vi "Unflatten LIDAR Data.vi"(11 "Flat LIDAR Data":dbl[](array[numeric])) -> (0 "Robot Pose x,y (m)":dbl[](array[numeric]), 1 "Robot Pose Theta (rad)":dbl, 2 "Bearing (rad)":dbl[](array[numeric]), 3 "Range (m)":dbl[](array[numeric]))   [LabVIEW 2017]
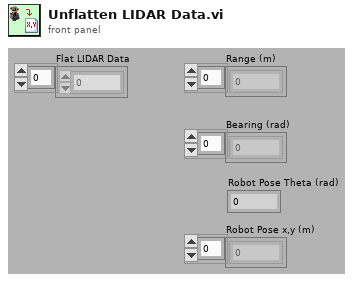
[diagram p1: front panel]
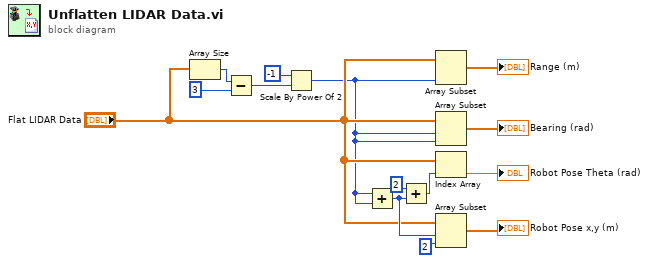
[diagram p0: block diagram]
diagram:
  n1 = Array Size(array="Flat LIDAR Data") -> (size(s)=w1:i32)
  n2 = Subtract(x=w1, y=3) -> (x-y=w3:i32)
  n3 = Scale By Power Of 2(n=-1, x=w3) -> (x*2^n=w5:i32)
  n4 = Add(x=w5, y=w5) -> (x+y=w11:i32)
  n5 = Add(x=2 ("y"), y=w11) -> (x+y=w9:i32)
  n6 = Array Subset(array="Flat LIDAR Data", length=w5) -> (→"Range (m)":dbl[])  [unwired: 1 in]
  n7 = Array Subset(array="Flat LIDAR Data", index=w5, length=w5) -> (→"Bearing (rad)":dbl[])
  n8 = Index Array(array="Flat LIDAR Data", index=w9) -> (element=→"Robot Pose Theta (rad)":dbl)
  n9 = Array Subset(array="Flat LIDAR Data", index=w11, length=2) -> (→"Robot Pose x,y (m)":dbl[])
